vi "Stop.vi"(8 "error in (no error)":errorcluster, 11 "2DArrayManager in":refnum<class "2DArrayManager.lvclass">) -> (0 "error out":errorcluster, 3 "2DArrayManager out":refnum<class "2DArrayManager.lvclass">)   [LabVIEW 2020, in "OOPanel.lvlib" / "2DArrayManager.lvclass"]
uses:
  2DArrayManager.lvclass
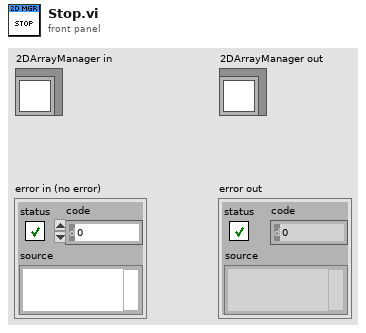
[diagram p1: front panel]
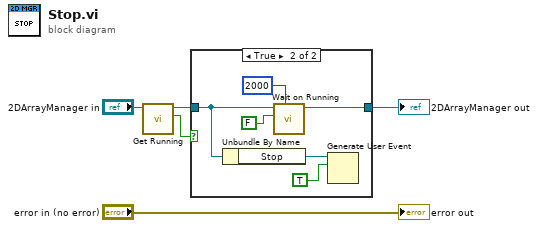
[diagram p0: block diagram]
diagram:
  n1 = call "Get Running.vi"("2DArrayManager in"="2DArrayManager in") -> ("Running"=w3:bool, "2DArrayManager out"=w4:refnum<class "2DArrayManager.lvclass">)  [unwired: 8 in, 1 out]
  n2 = case shown="True" w3 {
    tunnel: w4 -> [w6 w10]
    tunnel: [w6 w9] -> w1
    frame False {
    }
    frame True {
      n3 = Unbundle By Name(w10) -> ("Stop"=w12:refnum<user-event>)
      n4 = call "Wait on Running.vi"("Timeout (2000ms)"=2000, "Value"=FALSE, "2DArrayManager in"=w10) -> ("2DArrayManager out"=w9:refnum<class "2DArrayManager.lvclass">)  [unwired: 7 in, 1 out]
      n5 = Generate User Event(user event=w12, event data cluster=TRUE ("event data")) -> ()  [unwired: 2 in, 2 out]
    }
  }
  "2DArrayManager out" <- w1
  "error out" <- "error in (no error)"
